vi "Try Match Response.vi"(8 "error in":errorcluster, 10 "ICAN CC Frame":refnum<class "ICAN CC Frame.lvclass">, 11 "Upload Transfer in":refnum<class "Upload Transfer.lvclass">) -> (0 "error out":errorcluster, 1 "SDO Result":T1={"Success"=FALSE, "SDO abort code"={"Null"=TRUE, "Value"=84082688}, "Data"={"Null"=TRUE, "Data"=[]}} {"SDO abort code"."Value" items=["Toggle bit not allowed"=84082688, "SDO protocol timed out"=84148224, "Client/server command specifier not valid or unknown"=84148225, "Invalid block size (block mode only)"=84148226, "Invalid sequence number (block mode only)"=84148227, "CRC error (block mode only)"=84148228, "Out of memory"=84148229, "Attempt to read a write only object"=100728833, "Attempt to write a read only object"=100728834, "Object does not exist in the object dictionary"=100794368, "Object cannot be mapped to the PDO"=100925505, "The number and length of the objects to be mapped would exceed PDO length"=100925506, "General parameter incompatibility reason"=100925507, "General internal incompatibility in the device"=100925511, "Access failed due to an hardware error"=101056512, "Data type does not match, length of service parameter does not match"=101122064, "Data type does not match, length of service parameter too high"=101122066, "Data type does not match, length of service parameter too low"=101122067, "Sub-index does not exist"=101253137, "Invalid value for parameter (download only)"=101253168, "Value of parameter written too high (download only)"=101253169, "Value of parameter written too low (download only)"=101253170, "Maximum value is less than minimum value"=101253174, "Resource not available: SDO connection"=101318691, "General error"=134217728, "Data cannot be transferred or stored to the application"=134217760, "Data cannot be transferred or stored to the application because of local control"=134217761, "Data cannot be transferred or stored to the application because of the present device stable"=134217762, "Object dictionary dynamic generation fails or no object dictionary is present (e.g. object dictionary is generated from file and generation fails because of an file error)"=134217763, "No data available"=134217764]; "Data"."Data" format="%02x"}, 2 "Match":bool, 3 "SDO Transfer out":refnum<class "SDO Transfer.lvclass">)   [LabVIEW 2020, in "CANopen.lvlib" / "SDO Manager.lvlib" / "Upload Transfer.lvclass"]
uses:
  Upload Transfer.lvclass
  HAL/Source/Interfaces/ICAN CC Frame/ICAN CC Frame.lvclass
  SDO Transfer/SDO Transfer.lvclass
  Upload Transfer.lvclass/Upload Transfer.ctl
  D:/git/CANopen-LabVIEW/source/SDO Manager/SDO Manager/SDO Transfer/SDO Transfer.lvclass
  D:/git/CANopen-LabVIEW/source/SDO Manager/SDO Manager/Upload Transfer/Upload Transfer.lvclass
  CANopen Message/CANopen Message.lvclass
  SDO Transfer/SDO abort code.ctl
  Typedefs/SDO Result.ctl
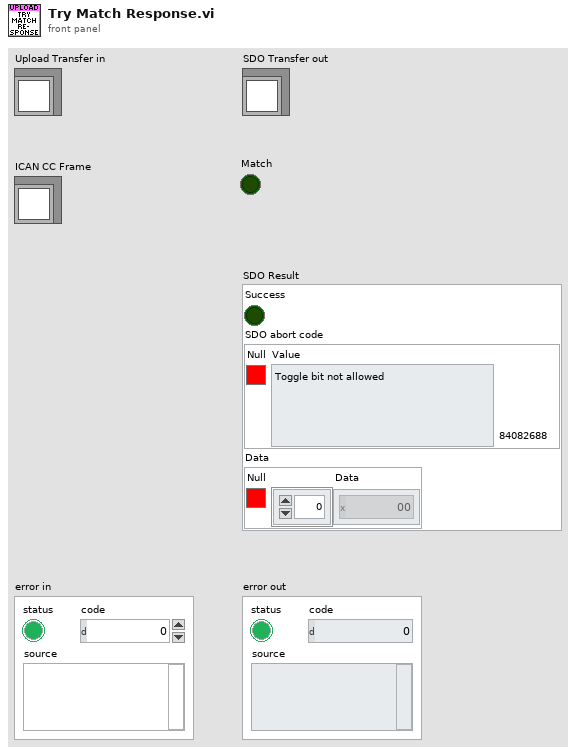
[diagram p1: front panel]
types:
  T1 = typedef "CANopen.lvlib/SDO Manager.lvlib/SDO Transfer.lvclass/SDO Result.ctl" = cluster{"Success":bool, "SDO abort code":cluster{"Null":bool, "Value":T2}, "Data":cluster{"Null":bool, "Data":u8[]}}
  T2 = typedef "CANopen.lvlib/SDO Manager.lvlib/SDO Transfer.lvclass/SDO abort code.ctl" = u32
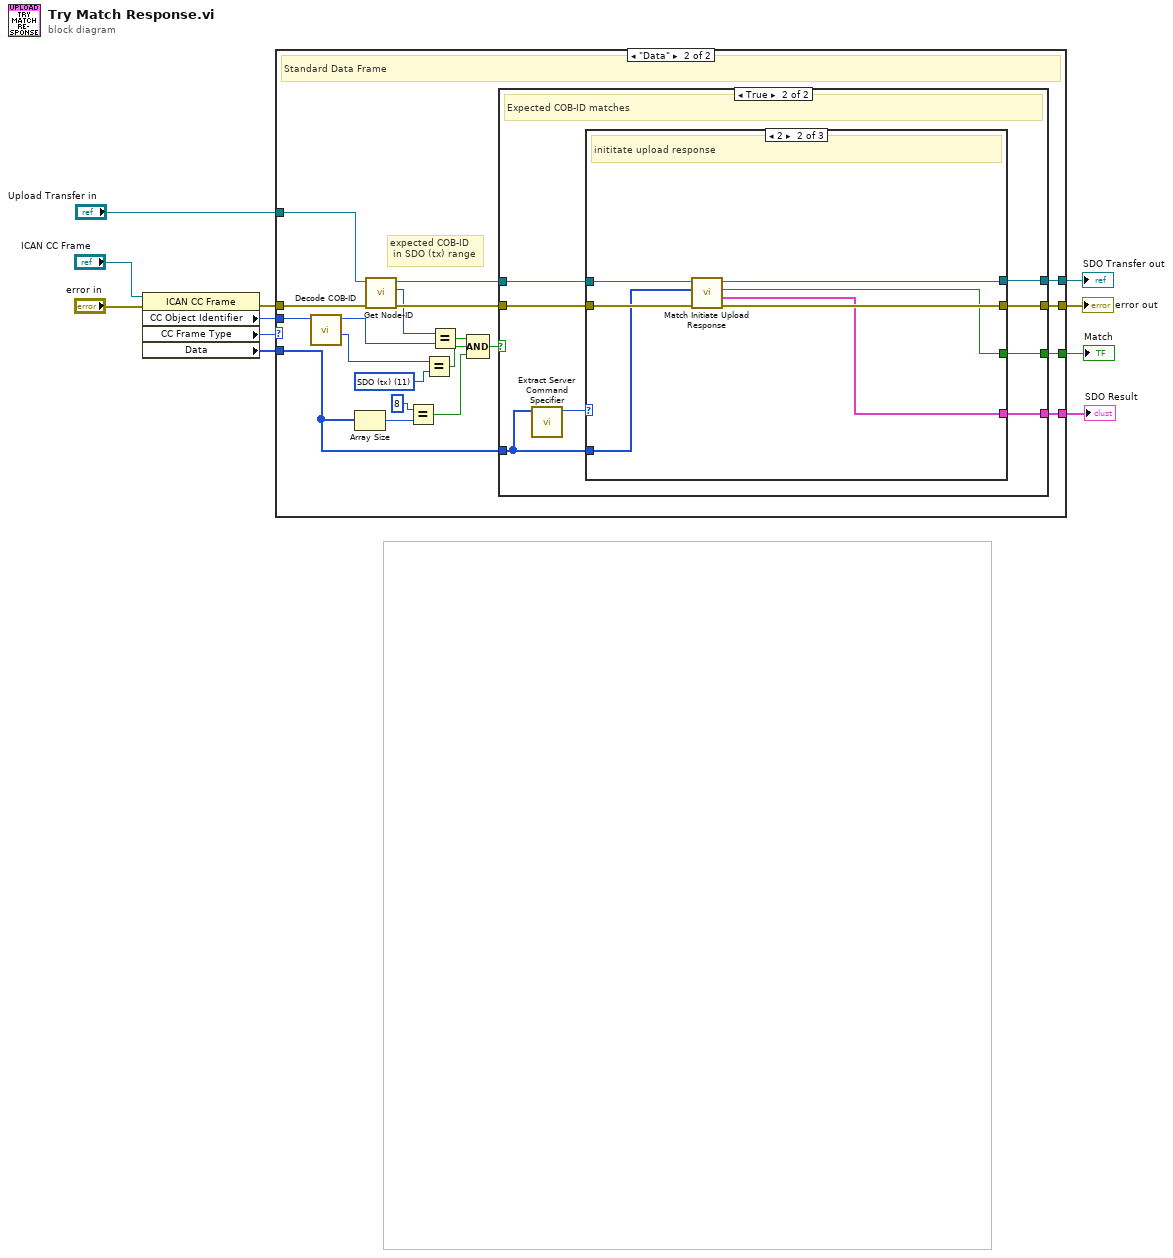
[diagram p0: block diagram]
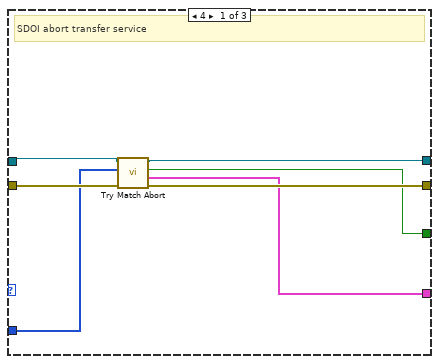
[diagram p4: hidden frame]
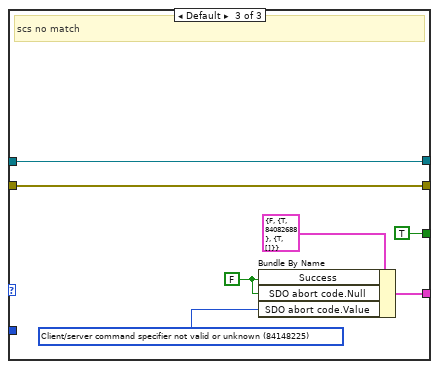
[diagram p5: hidden frame]
diagram:
  n1 = property class="ICAN CC Frame"(reference="ICAN CC Frame", error in="error in") -> (error out=w9:errorcluster, "CC Object Identifier"=w4:u32, "CC Frame Type"=w2:enum8{"Data", "Remote", "Error", "Overload"}, "Data"=w3:u8[])  [unwired: 1 out]
  n2 = case shown="\"Data\"" w2 {
    tunnel: w9 -> [w13 w33]
    tunnel: "Upload Transfer in" -> [w12 w32]
    tunnel: [w12 w29] -> w7
    tunnel: [w13 w28] -> w6
    tunnel: [_ w27] -> w5
    tunnel: w4 -> [_ w26]
    tunnel: w3 -> [_ w15]
    tunnel: [_ w14] -> w1
    frame Default {
      # "Wrong Frame Type"
    }
    frame "Data" {
      w23 = u8 11 items=["NMT"=0, "EMCY/SYNC"=1, "TIME"=2, "PDO1 (tx)"=3, "PDO1 (rx)"=4, "PDO2 (tx)"=5, "PDO2 (rx)"=6, "PDO3 (tx)"=7, "PDO3 (rx)"=8, "PDO4 (tx)"=9, "PDO4 (rx)"=10, "SDO (tx)"=11, "SDO (rx)"=12, "NMT error control"=14] ("Function Code")
      # "expected COB-ID\n in SDO (tx) range"
      # "Standard Data Frame"
      n3 = call "Decode COB-ID.vi"("COD-ID"=w26) -> ("Function Code"=w22:u8, "Node-ID"=w25:u8)  [unwired: 9 in]
      n4 = Array Size(array=w15) -> (size(s)=w21:i32)
      n5 = call "Get Node-ID.vi"("error in"=w33, "SDO Transfer in"=w32) -> ("error out"=w30:errorcluster, "Node-ID"=w24:u8, "SDO Transfer out"=w31:refnum<class "Upload Transfer.lvclass">)  [unwired: 7 in]
      n6 = Equal?(x=8, y=w21) -> (x = y?=w16:bool)
      n7 = Equal?(x=w22, y=w23) -> (x = y?=w17:bool)
      n8 = Equal?(x=w24, y=w25) -> (x = y?=w18:bool)
      n9 = Compound Arithmetic op=AND(w18, w17, w16) -> (w19:bool)
      n10 = case shown="True" w19 {
        tunnel: w31 -> [w35 w43]
        tunnel: w30 -> [w34 w42]
        tunnel: [w35 w39] -> w29
        tunnel: [w34 w40] -> w28
        tunnel: w15 -> [_ w37]
        tunnel: [_ w38] -> w27
        tunnel: [_ w36] -> w14
        frame False {
          # "no match"
        }
        frame True {
          # "Expected COB-ID matches"
          n11 = call "Extract Server Command Specifier.vi"("Data"=w37) -> ("Server Command Specifier"=w41:u8)  [unwired: 10 in]
          n12 = case shown="2" w41 {
            tunnel: w43 -> [w49 w55 w63]
            tunnel: w42 -> [w50 w57 w64]
            tunnel: [w46 w54 w63] -> w39
            tunnel: [w47 w56 w64] -> w40
            tunnel: [w45 w53 TRUE ("Match")] -> w38
            tunnel: w37 -> [w48 w52 _]
            tunnel: [w44 w51 w59] -> w36
            frame 4 {
              # "SDOI abort transfer service"
              n13 = call "Try Match Abort.vi"("error in"=w50, "Frame Data"=w48, "SDO Transfer in"=w49) -> ("error out"=w47:errorcluster, "SDO Result"=w44:T1, "Match"=w45:bool, "SDO Transfer out"=w46:refnum<class "Upload Transfer.lvclass">)  [unwired: 5 in]
            }
            frame 2 {
              # "inititate upload response"
              n14 = call "Match Initiate Upload Response.vi"("error in"=w57, "Frame Data"=w52, "SDO Transfer in"=w55) -> ("error out"=w56:errorcluster, "SDO Result"=w51:T1, "Match"=w53:bool, "SDO Transfer out"=w54:refnum<class "SDO Transfer.lvclass">)  [unwired: 5 in]
            }
            frame Default {
              w61 = FALSE ("Success")
              w60 = T2 84148225 items=["Toggle bit not allowed"=84082688, "SDO protocol timed out"=84148224, "Client/server command specifier not valid or unknown"=84148225, "Invalid block size (block mode only)"=84148226, "Invalid sequence number (block mode only)"=84148227, "CRC error (block mode only)"=84148228, "Out of memory"=84148229, "Attempt to read a write only object"=100728833, "Attempt to write a read only object"=100728834, "Object does not exist in the object dictionary"=100794368, "Object cannot be mapped to the PDO"=100925505, "The number and length of the objects to be mapped would exceed PDO length"=100925506, "General parameter incompatibility reason"=100925507, "General internal incompatibility in the device"=100925511, "Access failed due to an hardware error"=101056512, "Data type does not match, length of service parameter does not match"=101122064, "Data type does not match, length of service parameter too high"=101122066, "Data type does not match, length of service parameter too low"=101122067, "Sub-index does not exist"=101253137, "Invalid value for parameter (download only)"=101253168, "Value of parameter written too high (download only)"=101253169, "Value of parameter written too low (download only)"=101253170, "Maximum value is less than minimum value"=101253174, "Resource not available: SDO connection"=101318691, "General error"=134217728, "Data cannot be transferred or stored to the application"=134217760, "Data cannot be transferred or stored to the application because of local control"=134217761, "Data cannot be transferred or stored to the application because of the present device stable"=134217762, "Object dictionary dynamic generation fails or no object dictionary is present (e.g. object dictionary is generated from file and generation fails because of an file error)"=134217763, "No data available"=134217764] ("SDO abort code")
              # "scs no match"
              n15 = Bundle By Name(cluster=T1 {"Success"=FALSE, "SDO abort code"={"Null"=TRUE, "Value"=84082688}, "Data"={"Null"=TRUE, "Data"=[]}} ("SDO Result"), "Success"=w61, "SDO abort code.Null"=w61, "SDO abort code.Value"=w60) -> (w59:T1)
            }
          }
        }
      }
    }
  }
  "SDO Transfer out" <- w7
  "error out" <- w6
  "Match" <- w5
  "SDO Result" <- w1
